vi "StringToSSM.vi"(6 "Last Command (Stop)":string="Stop", 7 "Bus Reference":refnum<class "Bus.lvclass">, 8 "Error Out":errorcluster, 9 "Test Index (0)":i32, 10 "ModuleList":string[](array[string]), 11 "SSM Case":string="RunTest") -> (0 "Error Out 2":errorcluster, 2 "SSM Array":string[](array[string]))   [LabVIEW 2018]
doc: "This VI sends a message to loads the new plugin into the module."
uses:
  NistPluggableModules/BusClass/Bus.lvclass
  NistPluggableModules/BusClass/Bus.lvclass/Bus.ctl
  NistPluggableModules/BusClass/Accessors/Read Test.vi
  NistPluggableModules/TestClass/Test.lvclass
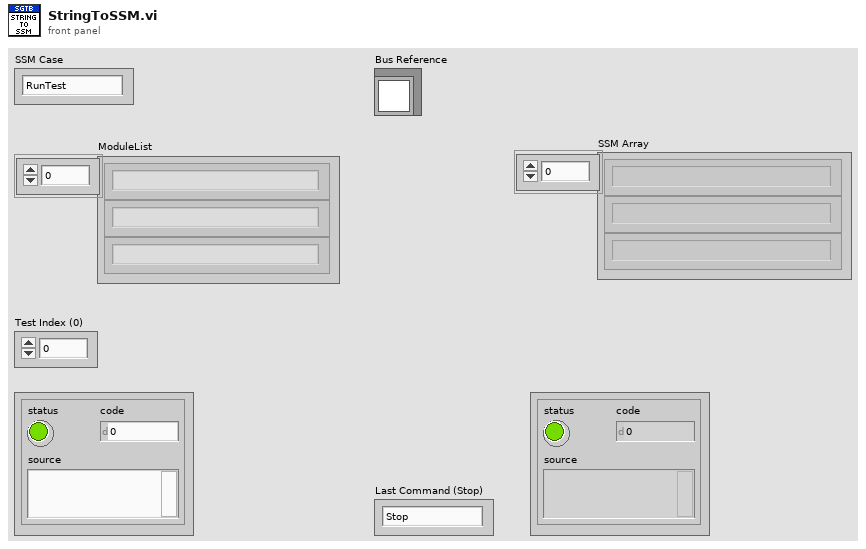
[diagram p1: front panel]
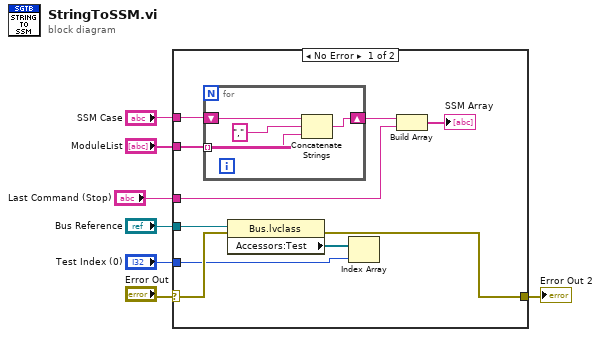
[diagram p0: block diagram]
diagram:
  n1 = case shown="No Error" "Error Out" {
    selector: "Error Out" -> [w12 w22]
    tunnel: "ModuleList" -> [w16 _]
    tunnel: "SSM Case" -> [w15 _]
    tunnel: [w9 w22] -> w4
    tunnel: "Test Index (0)" -> [w11 _]
    tunnel: "Bus Reference" -> [w10 _]
    tunnel: "Last Command (Stop)" -> [w8 _]
    frame No Error {
      n2 = for {
        tunnel: w16 -> [w18] mode=indexing
        shift-right: [w20] -> w17
        shift-left: w15 -> [w21]
        n3 = Concatenate Strings(w21, "," ("string"), w18) -> (w20:string)
      }
      n4 = property class="Bus.lvclass"(reference=w10, error in=w12) -> (error out=w9:errorcluster, "Accessors:Test"=w13:refnum<class "Test.lvclass">[])  [unwired: 1 out]
      n5 = Index Array(array=w13, index=w11) -> ()  [unwired: 1 out]
      n6 = Build Array(w17, w8) -> (→"SSM Array":string[])
    }
    frame Error {
    }
  }
  "Error Out 2" <- w4
